vi "Trasarea graficelor de functii utilizând noduri cu formule.vi"() -> ()   [LabVIEW 2011]
panel:
  out "XY Graph":cluster{i32[], dbl[]}(graph)
  in  "input X":dbl
  in  "input A":dbl
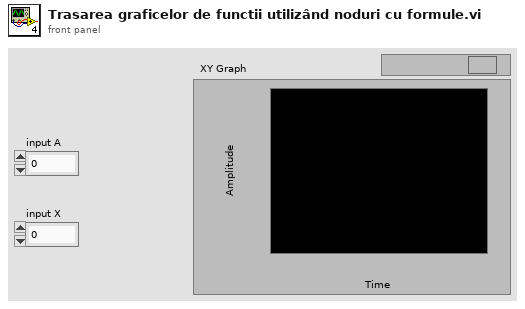
[diagram p1: front panel]
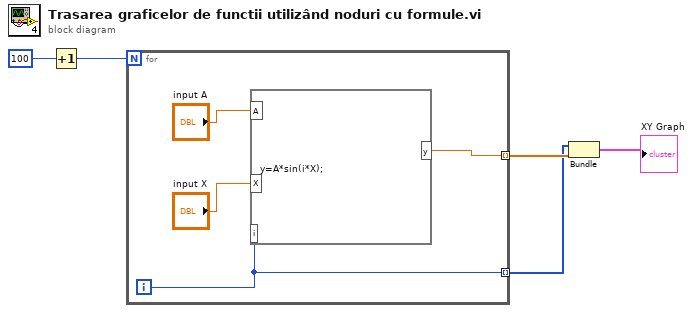
[diagram p0: block diagram]
diagram:
  n1 = Increment(x=100) -> (x+1=w4:i32)
  n2 = for {
    N: w4 -> [_]
    tunnel: [w7] -> w2 mode=indexing
    tunnel: [w6] -> w1 mode=indexing
    i -> [w6]
    n3 = formula code="y=A*sin(i*X);"("X"="input X", "A"="input A", "i"=w6) -> ("y"=w7:dbl)
  }
  n4 = Bundle "Bundle"(w1, w2) -> (→"XY Graph":cluster{i32[], dbl[]})  [unwired: 1 in]
